vi "System Semaphore Acquire.vi"(8 "error in (no error)":errorcluster, 10 "Timeout (ms)":u32=120000, 11 "SemaphoreHandle":u16 format="%.0x") -> (0 "error out":errorcluster, 2 "Iterations":i16, 3 "Timed Out?":bool)   [LabVIEW 2011]
uses:
  kernel32.dll
panel:
  out "Timeout":i16
  out "Semaphore Handle":i16 format="%x"
  out "Return Code":i16
  # "Acquires System Semaphore by Handle\n(Decreases Count by 1)"
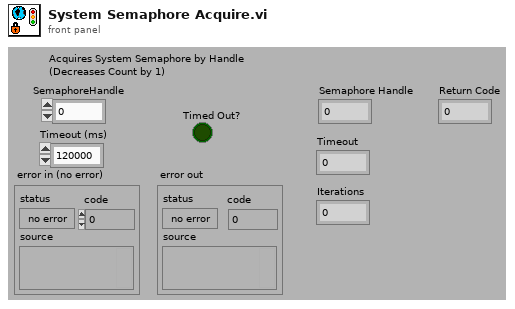
[diagram p1: front panel]
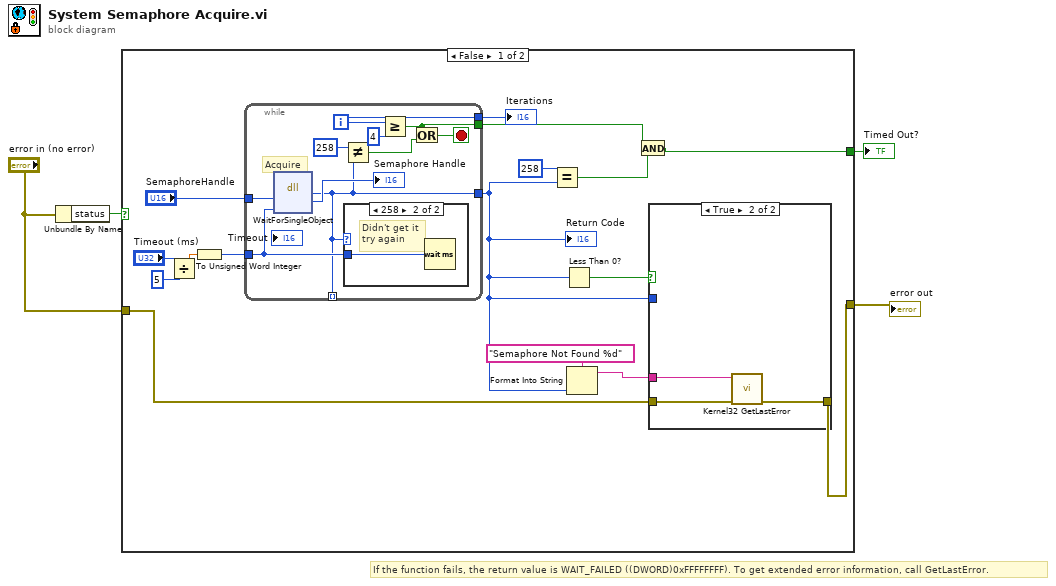
[diagram p0: block diagram]
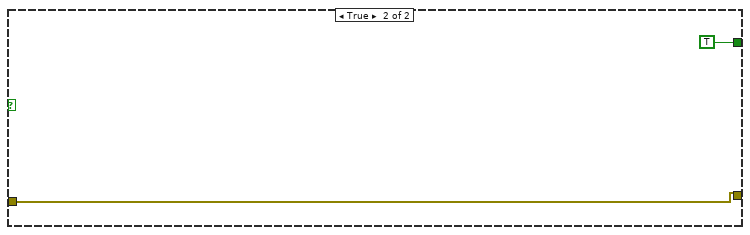
[diagram p4: hidden frame]
diagram:
  # "If the function fails, the return value is WAIT_FAILED ((DWORD)0xFFFFFFFF). To get extended error information, call GetLastError."
  n1 = Unbundle By Name("error in (no error)") -> ("status"=w4:bool)
  n2 = case shown="False" w4 {
    tunnel: "error in (no error)" -> [w19 w37]
    tunnel: [w18 w37] -> w2
    tunnel: [w9 TRUE] -> w1
    frame False {
      n3 = Divide(x="Timeout (ms)", y=u32 5 ("milliseconds to wait")) -> (x/y=w12:dbl)
      n4 = To Unsigned Word Integer(number=w12) -> (unsigned 16bit integer=w11:u16)
      n5 = while {
        tunnel: "SemaphoreHandle" -> [w30]
        tunnel: [w21] -> w7
        tunnel: w11 -> [w26]
        tunnel: [w23] -> w10
        tunnel: [w22] -> w8
        tunnel: [w21] -> _ mode=indexing
        i -> [w23]
        stop <- w27 stop-if-true
        # "Acquire"
        n6 = dll-call lib="kernel32.dll" fn="WaitForSingleObject"("SemaphoreHandle"=w30, "Timeoutms"=w26) -> (w21:i16, "SemaphoreHandle"=→"Semaphore Handle":u16)  [unwired: 4 in, 2 out]
        n7 = Not Equal?(x=i16 258, y=w21) -> (x != y?=w25:bool)
        n8 = case shown="258" w21 {
          tunnel: w26 -> [_ w31]
          frame Default {
            # "Acquired \nSemaphore\nKeep going"
          }
          frame 258 {
            # "Didn't get it\ntry again"
            n9 = Wait (ms)(milliseconds to wait=w31) -> ()  [unwired: 1 out]
          }
        }
        n10 = Greater Or Equal?(x=w23, y=u32 4 ("milliseconds to wait")) -> (x >= y?=w22:bool)
        n11 = Or(x=w22, y=w25) -> (x .or. y?=w27:bool)
      }
      "Return Code" <- w7
      "Iterations" <- w10
      n12 = Equal?(x=i16 258, y=w7) -> (x = y?=w5:bool)
      n13 = Less Than 0?(x=w7) -> (x < 0?=w17:bool)
      n14 = Format Into String(format string="Semaphore Not Found %d" ("source"), w7) -> (resulting string=w16:string)  [unwired: 2 in, 1 out]
      n15 = And(x=w8, y=w5) -> (x .and. y?=w9:bool)
      n16 = case shown="True" w17 {
        tunnel: w19 -> [w32 w35]
        tunnel: [w32 w34] -> w18
        tunnel: w7 -> [_ _]
        tunnel: w16 -> [_ w33]
        frame False {
          # "No Error"
        }
        frame True {
          n17 = call "Kernel32 GetLastError.vi"("error in (no error)"=w35, "Message"=w33) -> ("error out"=w34:errorcluster)  [unwired: 9 in]
        }
      }
    }
    frame True {
    }
  }
  "error out" <- w2
  "Timed Out?" <- w1
